vi "C4Hdl_reset.vi"(0 "c4hdl in":refnum<k24>, 11 "error in (no error)":errorcluster) -> (4 "c4hdl out":refnum<k24>, 15 "error out":errorcluster)   [LabVIEW 2015, in "libC4HdlLV.lvlib"]
uses:
  libC4HdlLV.lvlib
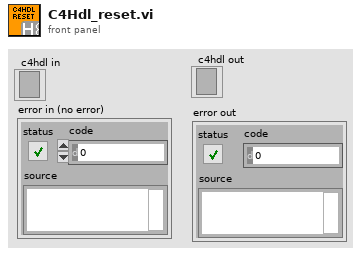
[diagram p1: front panel]
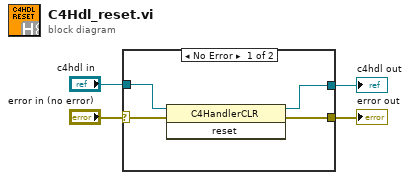
[diagram p0: block diagram]
diagram:
  n1 = case shown="No Error" "error in (no error)" {
    selector: "error in (no error)" -> [w6 w10]
    tunnel: [w8 w10] -> w4
    tunnel: [w7 w9] -> w3
    tunnel: "c4hdl in" -> [w5 w9]
    frame No Error {
      n2 = invoke class="C4HandlerCLR" method="reset"(reference=w5, error in=w6) -> (reference out=w7:refnum<k24>, error out=w8:errorcluster)  [unwired: 1 in, 1 out]
    }
    frame Error {
    }
  }
  "error out" <- w4
  "c4hdl out" <- w3
